vi "Scan.vi"(8 "error in (no error)":errorcluster, 11 "Scan Driver in":refnum<class "Scan Driver.lvclass">) -> (0 "error out":errorcluster, 2 "Again?":bool, 3 "Scan Driver out":refnum<class "Scan Driver.lvclass">)   [LabVIEW 2012, in "Scan Driver.lvclass"]
doc: "Main method for Scan Driver. Scan over the given Scanner, read data points from the given Readable, generate an onscreen graph, and write a data file."
uses:
  Scan Driver.lvclass
  Instruments/Utility Classes/Readable/X.ctl
  Scan Driver.lvclass/Scan Driver.ctl
  Scanners/Scanner/Scanner.lvclass
  Scan Graph.ctl
  File IO/File IO.lvclass
  Readers/Reader/Reader.lvclass
  Global/Misc.vi
  Global/Flags.vi
  Global/File Locations.vi
  Instruments/Utility Classes/Readable/Readable.lvclass
panel:
  out "?":string
  out "Data Monitor":cluster{"Name":string, "x":T1, "Unit":string}[](array[cluster])
  out "progress":string
  out "Time Estimate":string
  out "date":timestamp
  out "timedisp":string
  in  "log?":bool
  out "cpshigh":dbl caption="CPS High"
  in  "restart":bool
  out "busybar":bool[](array[boolean])
  out "done?":bool caption="Done"
  in  "Exit":bool
  in  "stop":bool
  in  "?":bool
  out "Primary Graph":T2(graph) caption="cpsgraph"
  out "time":dbl
  out "Secondary Graph":T2(graph)
  # "Log"
  # "Linear"
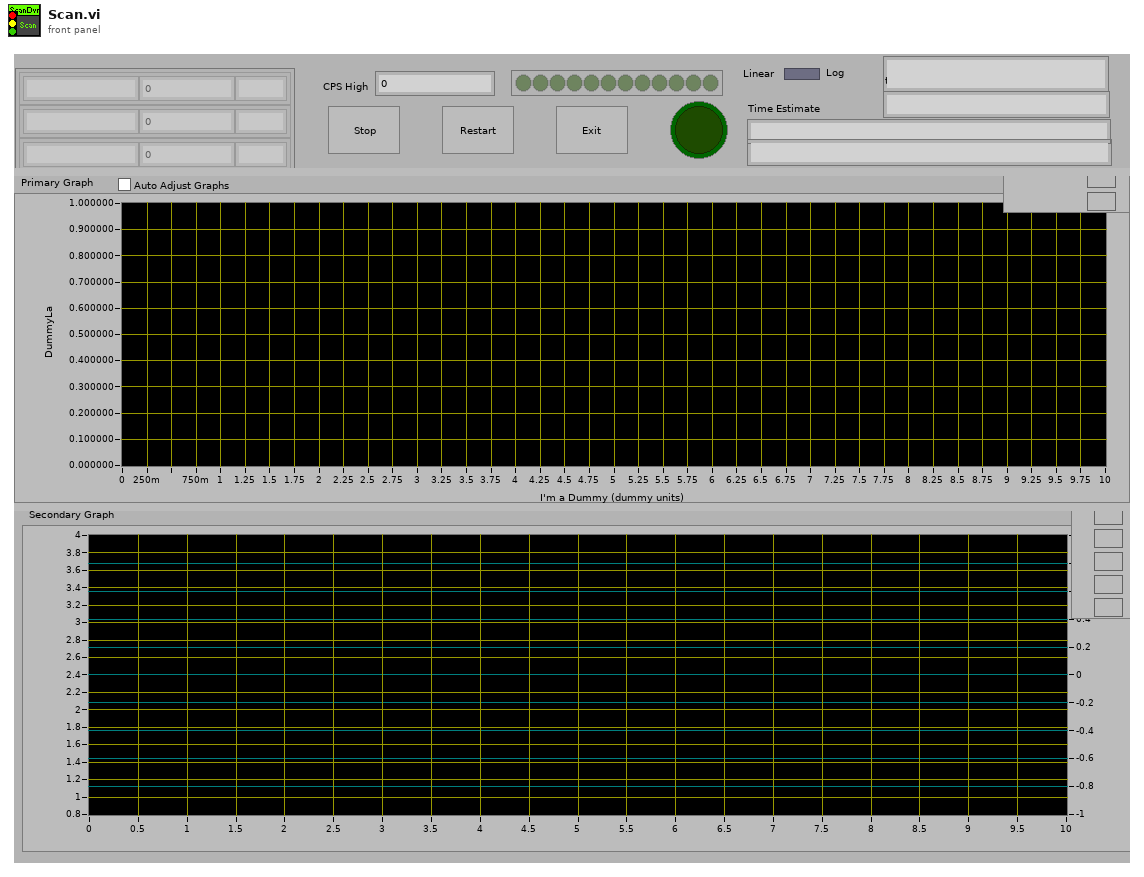
[diagram p1: front panel]
types:
  T1 = typedef "Readable.lvclass/X.ctl" = dbl
  T2 = typedef "Scan Driver.lvclass/Scan Graph.ctl" = cluster{"point array":cluster{"x":dbl, "y":dbl}[]}[]
  T3 = typedef "Scanner.lvclass/Range.ctl" = cluster{"xi":dbl, "xf":dbl, "dx":dbl, "Return to...?":bool, "Return to":dbl}
  T4 = typedef "Readable.lvclass/Data Channels.ctl" = T5[]
  T5 = typedef "Readable.lvclass/Data Channel.ctl" = cluster{"Name":string, "Data Point":T6, "Unit":string}
  T6 = typedef "Readable.lvclass/Data Point.ctl" = cluster{"t":T7, "x":T1}
  T7 = typedef "Readable.lvclass/Time.ctl" = timestamp
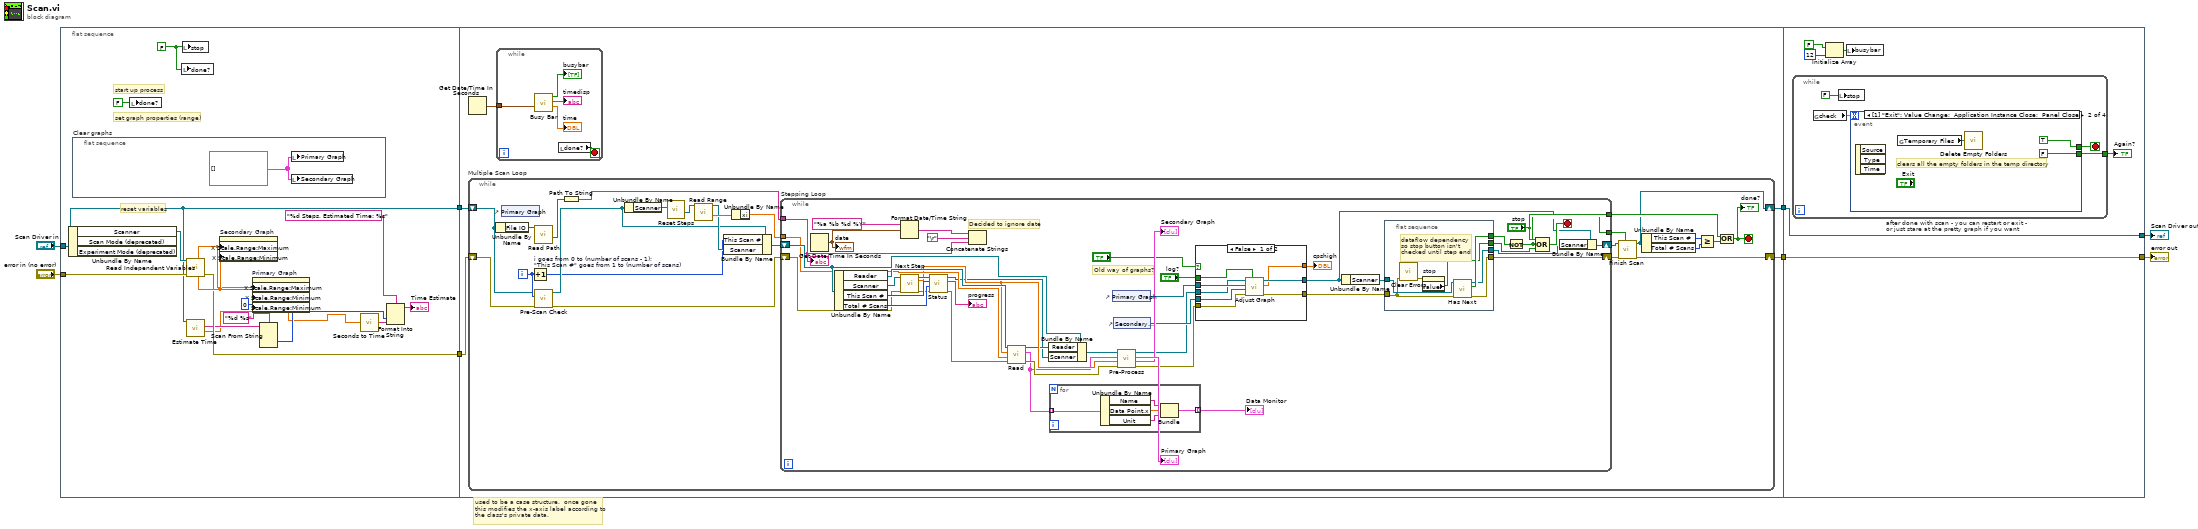
[diagram p0: block diagram]
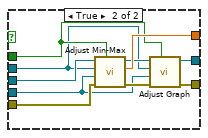
[diagram p2: hidden frame]
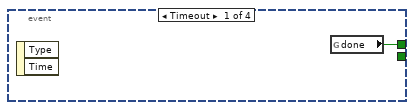
[diagram p3: hidden frame]
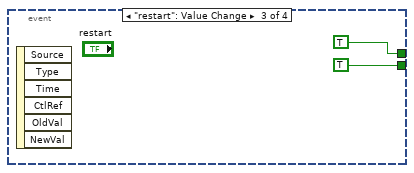
[diagram p4: hidden frame]
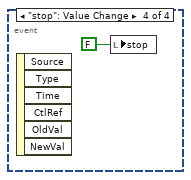
[diagram p5: hidden frame]
diagram:
  # "used to be a case structure.  once gone\nthis modifies the x-axis label according to\nthe class's private data."
  n1 = flat-sequence {
    tunnel: [w17] -> w4
    tunnel: [w21] -> w3
    tunnel: "error in (no error)" -> [w20]
    tunnel: "Scan Driver in" -> [w17]
    tunnel: w4 -> [w29]
    tunnel: [w28] -> w2
    tunnel: w3 -> [w27]
    tunnel: [w26] -> w1
    tunnel: [w135] -> w8
    tunnel: [w134] -> w5
    tunnel: w2 -> [w135]
    tunnel: w1 -> [w134]
    frame #0 {
      w19 = FALSE
      # "reset variables"
      # "start up process"
      # "set graph properties (range)"
      n2 = Unbundle By Name(w17) -> ("Scanner"=w18:refnum<class "Scanner.lvclass">)  [unwired: 2 out]
      n3 = flat-sequence "Clear graphs" {
        frame #0 {
          w25 = T2 []
          n4 = local write "Primary Graph"(w25) -> ()
          n5 = local write "Secondary Graph"(w25) -> ()
        }
      }
      n6 = local write "done?"(FALSE) -> ()
      n7 = local write "done?"(w19) -> ()
      n8 = local write "stop"(w19) -> ()
      n9 = call-dynamic "Read Independent Variables.vi"("error in (no error)"=w20, "Scanner.lvclass in"=w18) -> ("error out"=w21:errorcluster, "min value"=w24:dbl, "max value"=w23:dbl)  [unwired: 7 out]
      n10 = call "Estimate Time.vi"("Scan Driver in"=w17) -> ("Seconds"=w9:dbl[unit], "Time Estimate"=w15:string)  [unwired: 1 in, 8 out]
      n11 = property on="Secondary Graph" class="XYGraph (strict)"("X Scale.Range:Maximum"=w23, "X Scale.Range:Minimum"=w24) -> ()  [unwired: 2 in, 2 out]
      n12 = property on="Primary Graph" class="XYGraph (strict)"("X Scale.Range:Maximum"=w23, "X Scale.Range:Minimum"=w24, "Y Scale.Range:Minimum"=0) -> ()  [unwired: 2 in, 2 out]
      n13 = Scan From String(format string="%d %s", input string=w15) -> (output 1=w12:i32)  [unwired: 5 in, 3 out]
      n14 = call "Seconds to Time.vi"("Seconds"=w9) -> ("Time"=w11:string)
      n15 = Format Into String(format string="%d Steps, Estimated Time: %s", w12, w11) -> (resulting string=→"Time Estimate":string)  [unwired: 2 in, 1 out]
    }
    frame #1 {
      n16 = Get Date/Time In Seconds() -> (seconds since 1Jan1904=w30:timestamp)
      n17 = while "Multiple Scan Loop" {
        shift-right: [w51] -> w28
        shift-left: w29 -> [w40]
        shift-right: [w54] -> w26
        shift-left: w27 -> [w50]
        i -> [w42]
        stop <- w58 stop-if-true
        n18 = Unbundle By Name(w40) -> ("File IO"=w39:refnum<class "File IO.lvclass">)
        n19 = control-ref of="Primary Graph"() -> ()  [unwired: 1 out]
        n20 = Increment "i goes from 0 to (number of scans - 1);\n\"This Scan #\" goes from 1 to (number of scans)"(x=w42) -> (x+1=w43:i32)
        n21 = call-dynamic "Read Path.vi"("File IO.lvclass in"=w39) -> ("File Path"=w38:path)  [unwired: 6 in, 4 out]
        n22 = call "Pre-Scan Check.vi"("error in (no error)"=w50, "Current scan #"=w42, "Scan Driver in"=w40) -> ("error out"=w49:errorcluster, "Scan Driver out"=w44:refnum<class "Scan Driver.lvclass">)  [unwired: 2 in, 5 out]
        n23 = Path To String(path=w38) -> (string=w37:string)
        n24 = Unbundle By Name(w44) -> ("Scanner"=w46:refnum<class "Scanner.lvclass">)
        n25 = call "Reset Steps.vi"("Scanner.lvclass"=w46) -> ("Scanner.lvclass"=w36:refnum<class "Scanner.lvclass">)  [unwired: 10 in]
        n26 = call-dynamic "Read Range.vi"("Scanner.lvclass in"=w36) -> ("Range"=w48:T3, "Scanner.lvclass out"=w47:refnum<class "Scanner.lvclass">)  [unwired: 1 in, 8 out]
        n27 = Bundle By Name(cluster=w44, "This Scan #"=w43, "Scanner"=w47) -> (w45:refnum<class "Scan Driver.lvclass">)
        n28 = Unbundle By Name(w48) -> ("xi"=w41:dbl)
        n29 = while "Stepping Loop" {
          tunnel: ["stop"] -> w60
          shift-right: [w89] -> w55
          shift-left: w45 -> [w84]
          shift-right: [w92] -> w56
          shift-left: w49 -> [w86]
          tunnel: [w95] -> w53
          tunnel: w41 -> [w81]
          tunnel: w37 -> [w61]
          stop <- w103 stop-if-true
          # "Old way of graphs?"
          # "Decided to ignore date"
          n30 = Get Date/Time In Seconds() -> (seconds since 1Jan1904=w75:timestamp)
          "date" <- w75
          n31 = Unbundle By Name(w84) -> ("Reader"=w83:refnum<class "Reader.lvclass">, "Scanner"=w85:refnum<class "Scanner.lvclass">, "This Scan #"=w94:u32, "Total # Scans"=w97:u32)
          n32 = Format Date/Time String(time format string (%c)="%a %b %d %Y", seconds (now)=w75) -> (date/time string=w73:string)  [unwired: 1 in]
          n33 = call-dynamic "Next Step.vi"("error in (no error)"=w86, "Scanner in"=w85) -> ("error out"=w87:errorcluster, "Current Position"=w80:dbl, "Scanner out"=w88:refnum<class "Scanner.lvclass">)  [unwired: 7 out]
          n34 = call-dynamic "Status.vi"("error in (no error)"=w87, "totalscans"=w97, "scan#"=w94, "Scanner.lvclass in"=w88) -> ("error out"=w82:errorcluster, "scanprogress"=→"progress":string, "Scanner.lvclass out"=w71:refnum<class "Scanner.lvclass">)  [unwired: 5 out]
          n35 = Concatenate Strings(w73, "\r", w61) -> ()  [unwired: 1 out]
          n36 = call-dynamic "Read.vi"("error in (no error)"=w82, "Starting independent variable"=w81, "Current independent variable"=w80, "Reader in"=w83) -> ("error out"=w99:errorcluster, "Data Channels"=w78:T4, "Reader out"=w79:refnum<class "Reader.lvclass">)  [unwired: 5 out]
          n37 = Bundle By Name(cluster=w84, "Reader"=w79, "Scanner"=w71) -> (w98:refnum<class "Scan Driver.lvclass">)
          n38 = for {
            tunnel: w78 -> [w133] mode=indexing
            tunnel: [w129] -> w77 mode=indexing
            n39 = Unbundle By Name(w133) -> ("Name"=w130:string, "Data Point.x"=w131:T1, "Unit"=w132:string)
            n40 = Bundle("Name"=w130, "x"=w131, "Unit"=w132) -> (w129:cluster{"Name":string, "x":T1, "Unit":string})  [unwired: 1 in]
          }
          "Data Monitor" <- w77
          n41 = control-ref of="Primary Graph"() -> (w70:refnum<vi>)
          n42 = control-ref of="Secondary Graph"() -> (w69:refnum<vi>)
          n43 = call "Pre-Process.vi"("error in"=w99, "Actual X position"=w80, "New Data Points"=w78, "Scan Driver.lvclass in"=w98) -> ("error out"=w67:errorcluster, "Secondary Graph"=→"Secondary Graph":T2, "Primary Graph"=→"Primary Graph":T2, "Scan Driver.lvclass out"=w68:refnum<class "Scan Driver.lvclass">)  [unwired: 3 in, 1 out]
          n44 = case shown="False" "?" {
            tunnel: w70 -> [w111 w113]
            tunnel: w69 -> [w110 w112]
            tunnel: w68 -> [w109 w121]
            tunnel: w67 -> [w108 w120]
            tunnel: [w104 w117] -> w66
            tunnel: [w106 w118] -> w65
            tunnel: [w105 w119] -> w64
            tunnel: "log?" -> [w107 w114]
            frame False {
              n45 = call "Adjust Graph.vi"("log?"=w107, "error in (no error)"=w108, "Secondary Graph"=w110, "Primary Graph"=w111, "Scan Driver.lvclass"=w109) -> ("error out"=w104:errorcluster, "High"=w105:dbl, "Scan Driver.lvclass out"=w106:refnum<class "Scan Driver.lvclass">)  [unwired: 4 in]
            }
            frame True {
              n46 = call "Adjust Min-Max.vi"("log?"=w114, "error in (no error)"=w120, "Secondary Graph"=w112, "Primary Graph"=w113, "Scan Driver.lvclass"=w121) -> ("error out"=w116:errorcluster, "High"=w119:dbl, "Scan Driver.lvclass out"=w115:refnum<class "Scan Driver.lvclass">)  [unwired: 3 in, 1 out]
              n47 = call "Adjust Graph.vi"("log?"=w114, "error in (no error)"=w116, "Secondary Graph"=w112, "Primary Graph"=w113, "Scan Driver.lvclass"=w115) -> ("error out"=w117:errorcluster, "Scan Driver.lvclass out"=w118:refnum<class "Scan Driver.lvclass">)  [unwired: 4 in, 1 out]
            }
          }
          "cpshigh" <- w64
          n48 = Unbundle By Name(w65) -> ("Scanner"=w91:refnum<class "Scanner.lvclass">)
          n49 = flat-sequence {
            tunnel: [w128] -> w93
            tunnel: w66 -> [w123]
            tunnel: [w127] -> w92
            tunnel: w91 -> [w126]
            tunnel: [w125] -> w90
            tunnel: [w122] -> w76
            frame #0 {
              # "dataflow dependency\nso stop button isn't\nchecked until step end"
              n50 = call <vilib>:"Clear Errors.vi"("error in (no error)"=w123) -> ("error out"=w124:errorcluster)  [unwired: 6 in]
              n51 = property on="stop" class="Bool (strict)"(error in=w124) -> ("Value"=w122:bool)  [unwired: 1 in, 2 out]
              n52 = call-dynamic "Has Next.vi"("error in (no error)"=w123, "Scanner.lvclass in"=w126) -> ("error out"=w127:errorcluster, "Again?"=w128:bool, "Scanner.lvclass out"=w125:refnum<class "Scanner.lvclass">)  [unwired: 7 out]
            }
          }
          n53 = Not(x=w93) -> (.not. x?=w95:bool)
          n54 = Compound Arithmetic op=OR("stop", w95, w76) -> (w103:bool)
          n55 = Bundle By Name(cluster=w65, "Scanner"=w90) -> (w89:refnum<class "Scan Driver.lvclass">)
          "?" <- w61
        }
        n56 = call "Finish Scan.vi"("Scan finished successfully?"=w53, "error in"=w56, "Scan Driver.lvclass in"=w55) -> ("error out"=w54:errorcluster, "Scan Driver.lvclass out"=w51:refnum<class "Scan Driver.lvclass">)  [unwired: 2 in, 5 out]
        n57 = Unbundle By Name(w51) -> ("This Scan #"=w52:u32, "Total # Scans"=w57:u32)
        n58 = Greater Or Equal?(x=w52, y=w57) -> (x >= y?=w59:bool)
        n59 = Compound Arithmetic op=OR(w60, w59) -> (w58:bool)
        "done?" <- w58
      }
      n60 = while {
        tunnel: w30 -> [w34]
        stop <- w33 stop-if-true
        n61 = call "Busy Bar.vi"("basetime"=w34) -> ("Elapsed Seconds"=→"time":dbl, "Time"=→"timedisp":string, "Busy Bar"=→"busybar":bool[])  [unwired: 1 in, 7 out]
        n62 = local read "done?"() -> (w33:bool)
      }
    }
    frame #2 {
      n63 = while "after done with scan - you can restart or exit - or just stare at the pretty graph if you want" {
        tunnel: [w141] -> w136
        stop <- w140 stop-if-true
        n64 = global read "Misc.vi" "check"() -> (w142:dbl)
        n65 = local write "stop"(FALSE ("stop")) -> ()
        n66 = event shown="[1] \"Exit\": Value Change;  Application Instance Close;  Panel Close" {
          selector: _ -> [_ _ _ _]
          dyn-events: _ -> [_ _ _ _]
          timeout: w142 -> [_ _ _ _]
          tunnel: [w144 TRUE TRUE ("done") _] -> w140
          tunnel: [_ FALSE TRUE ("done") _] -> w141
          event Timeout {
            n67 = event-data() -> ()  [unwired: 3 out]
            n68 = global read "Flags.vi" "done"() -> (w144:bool)
          }
          event "Exit": Value Change; Application Instance Close; Panel Close {
            # "clears all the empty folders in the temp directory"
            n69 = event-data() -> ()  [unwired: 4 out]
            n70 = global read "File Locations.vi" "Temporary Files"() -> (w146:path)
            n71 = call "Delete Empty Folders.vi"("dirpath"=w146) -> ()  [unwired: 5 out]
          }
          event "restart": Value Change {
            n72 = event-data() -> ()  [unwired: 7 out]
          }
          event "stop": Value Change {
            n73 = event-data() -> ()  [unwired: 7 out]
            n74 = local write "stop"(FALSE) -> ()
          }
        }
      }
      "Again?" <- w136
      n75 = Initialize Array(FALSE, 12) -> (w139:bool[])
      n76 = local write "busybar"(w139) -> ()
    }
  }
  "Scan Driver out" <- w8
  "error out" <- w5
